vi "Varient_Creator.vi"(8 "error in (no error)":errorcluster) -> (0 "error out":errorcluster)   [LabVIEW 2017]
uses:
  <vilib>/Utility/file.llb/Read Delimited Spreadsheet (string).vi
  <vilib>/Utility/file.llb/Write Delimited Spreadsheet (string).vi
  557cc533-a4ba-4953-a7b5-ba01b5e60265.vi
panel:
  in  "Varient Details":string[][](table)
  in  "Test Resistor":string(combo)
  in  "Magnetic Asyl":string(combo)
  in  "Kinematic Asyl":string(combo)
  in  "CBCT Group":string(combo)
  in  "PMR":string(combo)
  in  "Hausing No":string(combo)
  in  "Delete Button":bool
  in  "Save Button":bool
  in  "Sr  No":u16=1 min=1 max=100 step=1
  in  "HOME":bool
  in  "UPDATE TABLE":bool
  in  "FG CAT No":string(combo)
  # "Varient Creater"
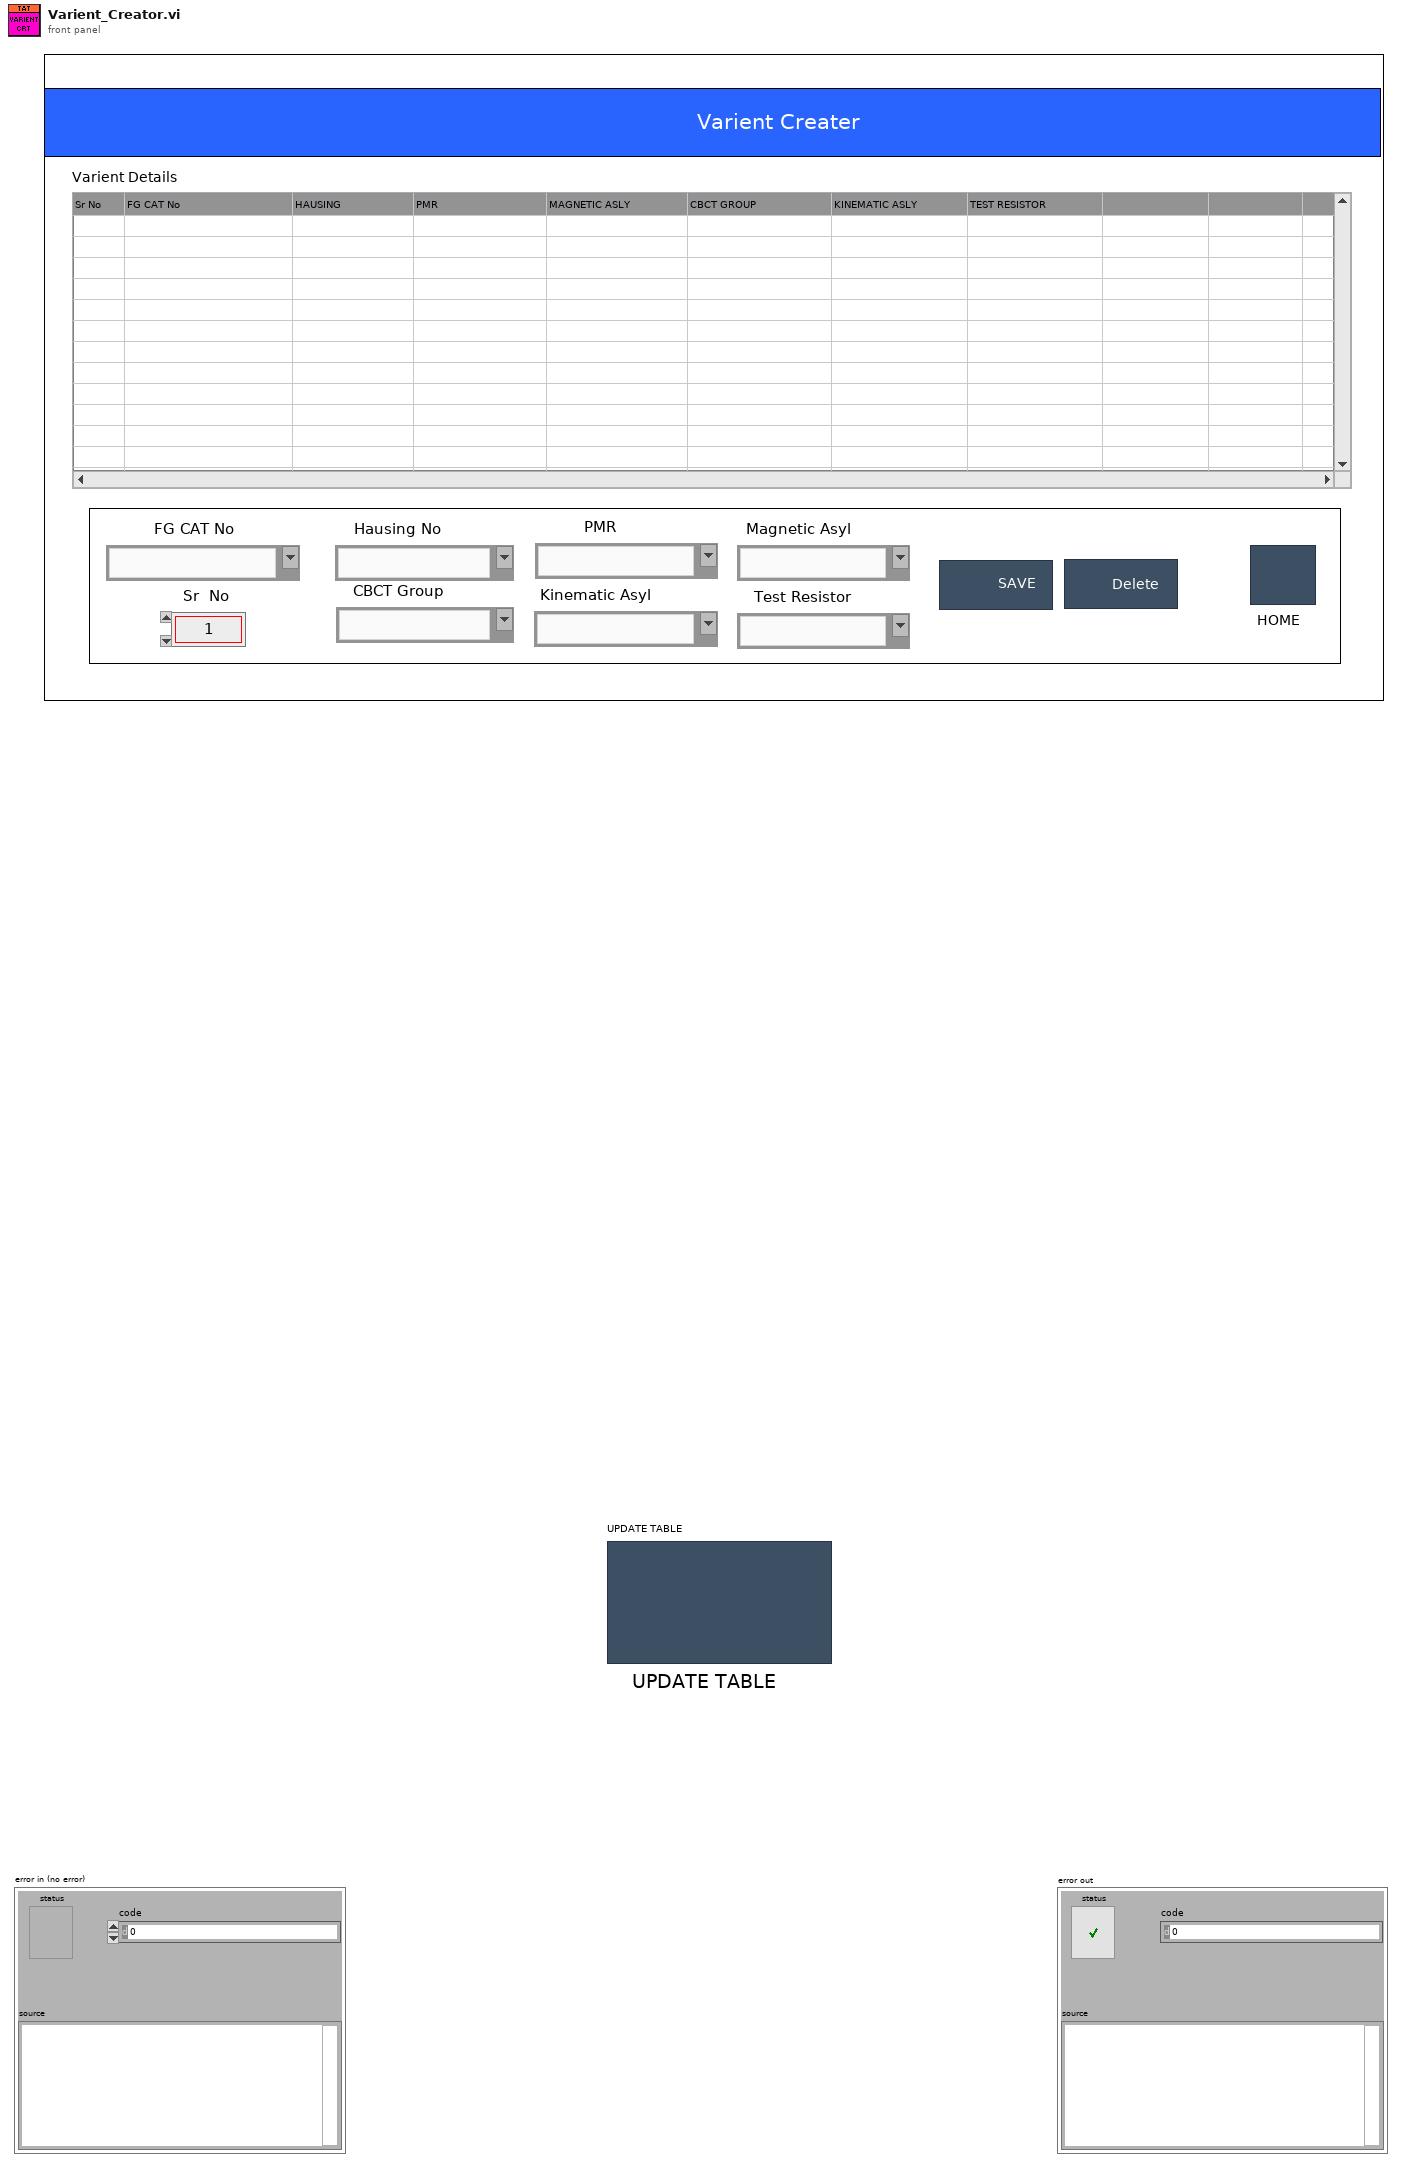
[diagram p1: front panel]
types:
  T1 = enum32{"invalid app kind", "Development System", "Run Time System", "Student Edition", "Embedded LabVIEW", "Evaluation", "Custom"}
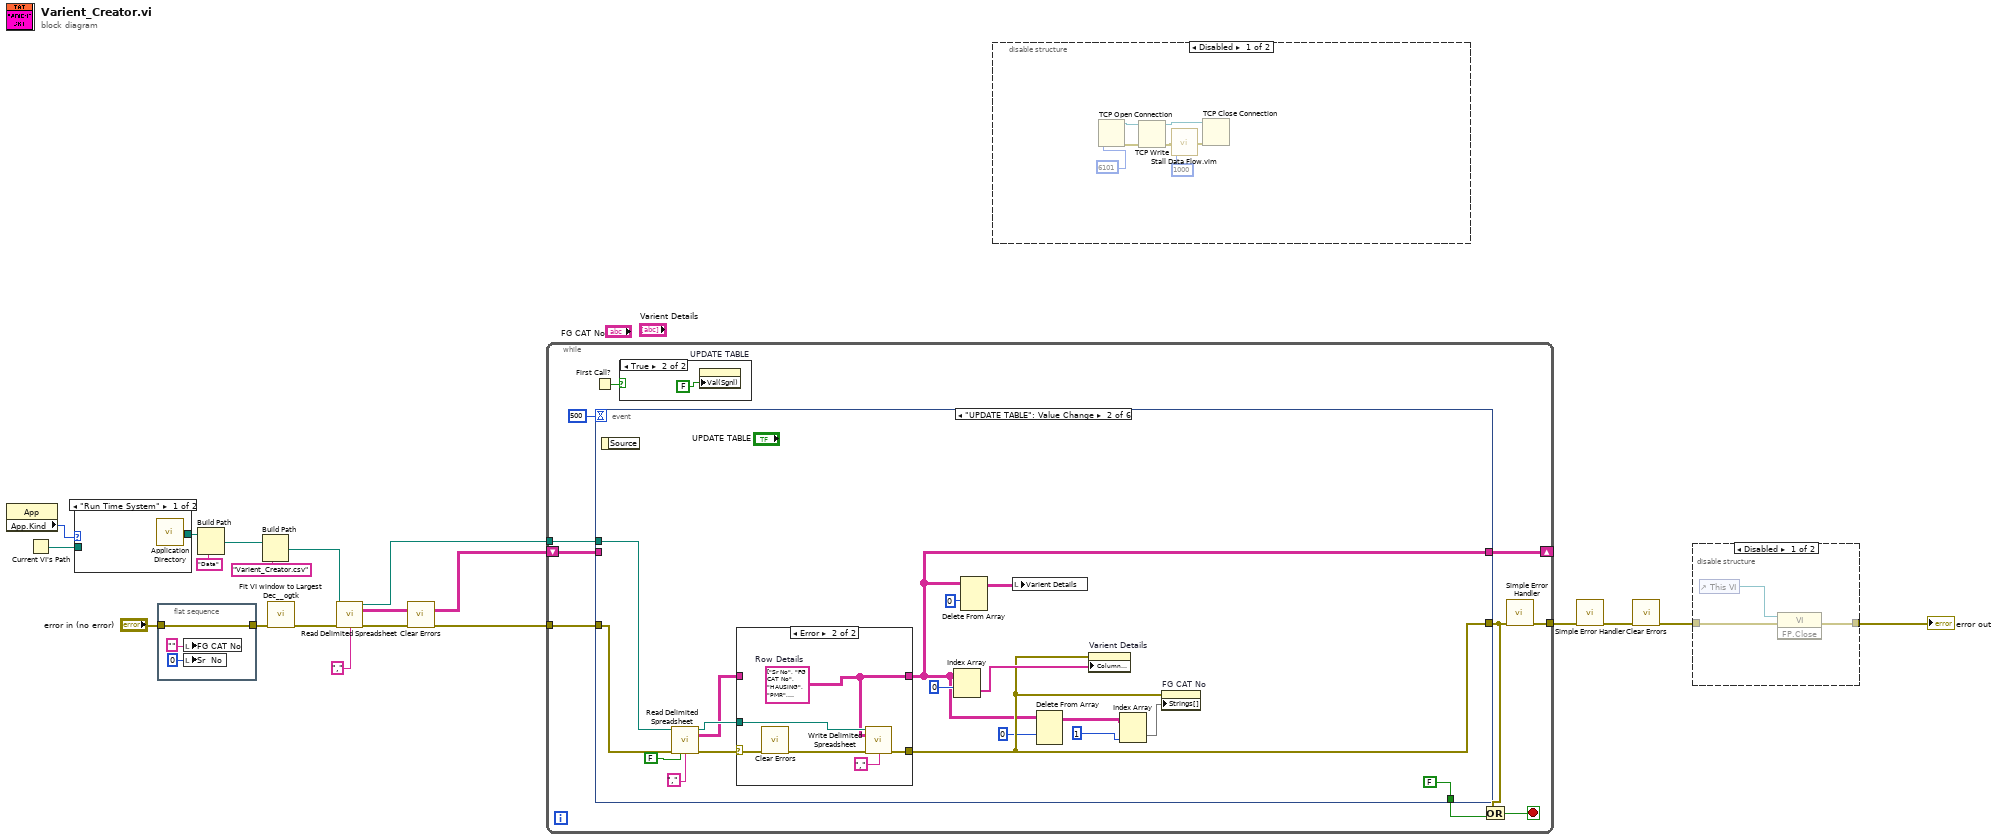
[diagram p0: block diagram]
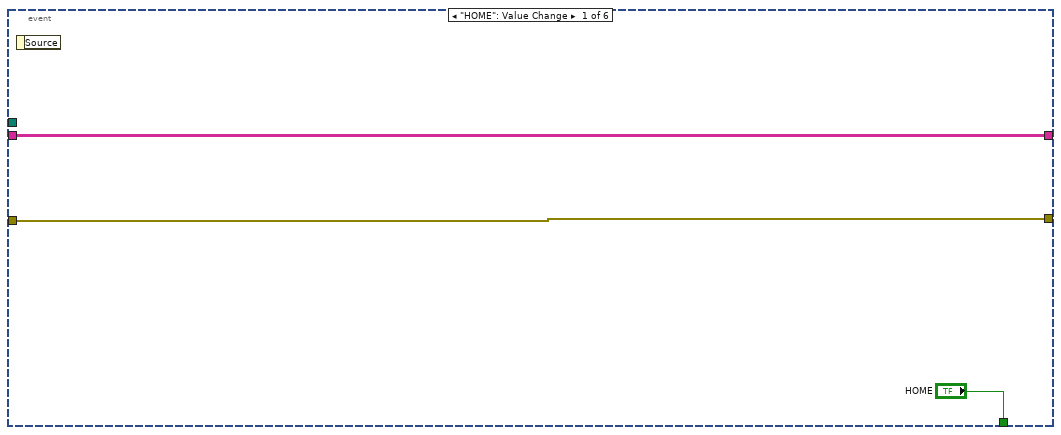
[diagram p3: hidden frame]
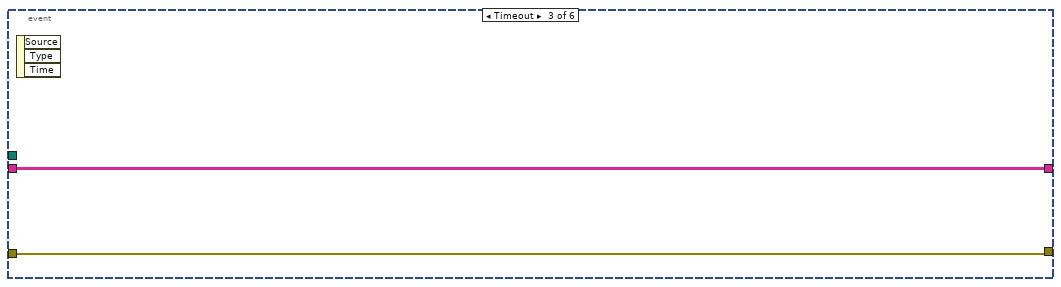
[diagram p5: hidden frame]
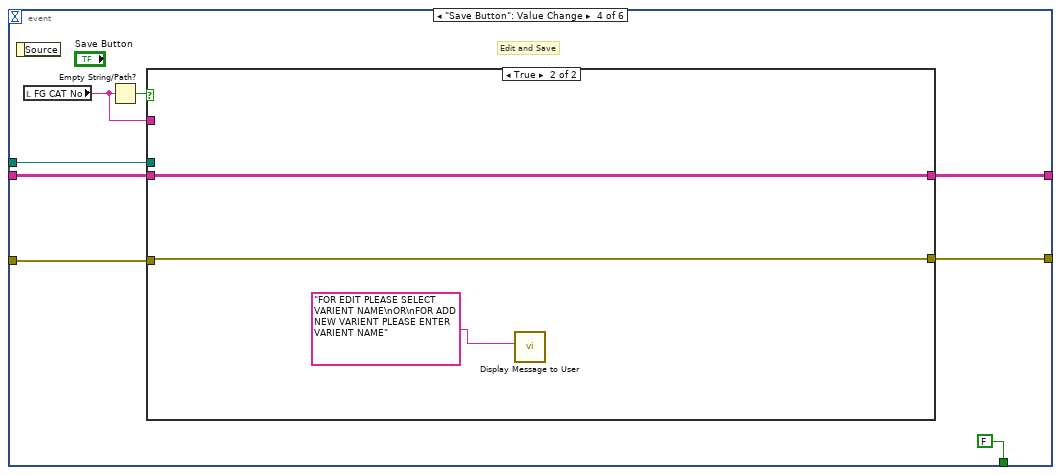
[diagram p6: hidden frame]
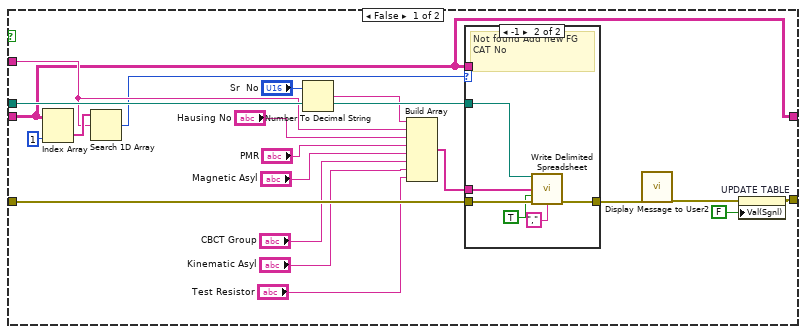
[diagram p7: hidden frame]
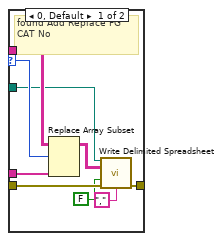
[diagram p8: hidden frame]
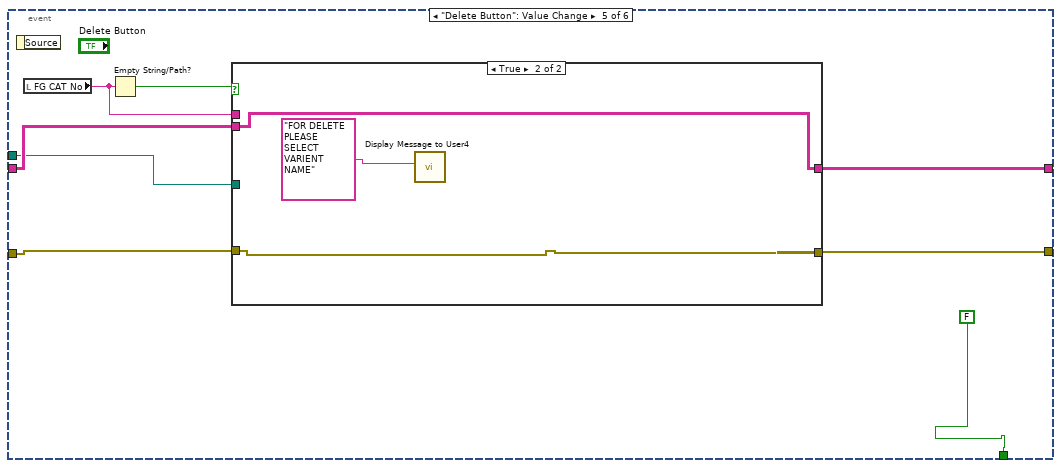
[diagram p9: hidden frame]
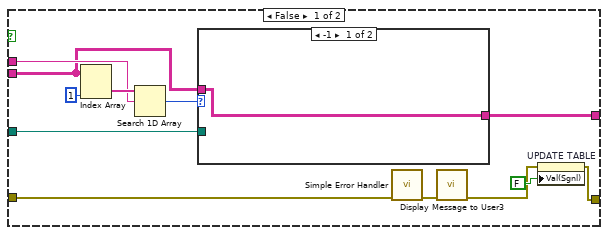
[diagram p10: hidden frame]
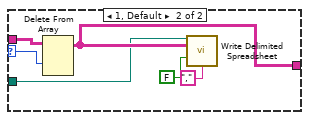
[diagram p11: hidden frame]
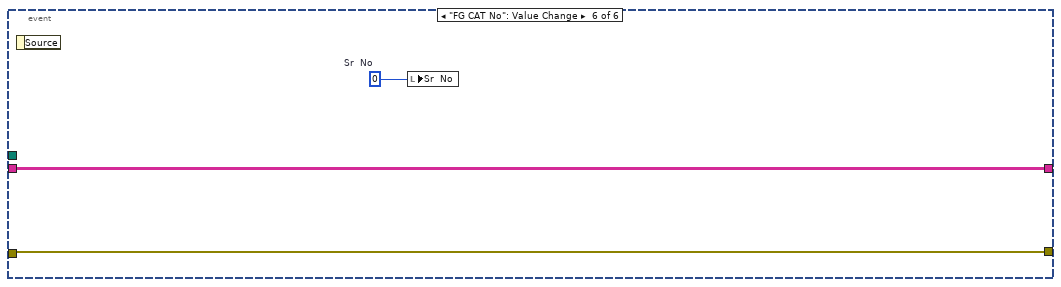
[diagram p12: hidden frame]
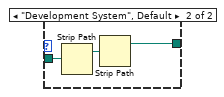
[diagram p15: hidden frame]
diagram:
  n1 = property class="App"() -> ("App.Kind"=w12:T1)  [unwired: 2 in, 2 out]
  n2 = Current VI's Path() -> (path=w13:path)
  n3 = case shown="\"Run Time System\"" w12 {
    tunnel: w13 -> [_ w22]
    tunnel: [w20 w21] -> w9
    frame "Run Time System" {
      n4 = call <vilib>:"Application Directory.vi"() -> ("Application Directory"=w20:path)
    }
    frame "Development System", Default {
      n5 = Strip Path(path=w22) -> (stripped path=w23:path)  [unwired: 1 out]
      n6 = Strip Path(path=w23) -> (stripped path=w21:path)  [unwired: 1 out]
    }
  }
  n7 = flat-sequence {
    tunnel: [w26] -> w14
    tunnel: "error in (no error)" -> [w26]
    frame #0 {
      n8 = local write "FG CAT No"("" ("PART NUMBER")) -> ()
      n9 = local write "Sr  No"(u16 0 ("BATCH SIZE")) -> ()
    }
  }
  n10 = Build Path(base path=w9, name or relative path="Data") -> (appended path=w10:path)
  n11 = Build Path(base path=w10, name or relative path="Varient_Creator.csv") -> (appended path=w1:path)
  n12 = call <userlib>:"Fit VI window to Largest Dec__ogtk.vi"("error in (no error)"=w14) -> ("error out"=w6:errorcluster)  [unwired: 5 in, 1 out]
  n13 = call-poly <vilib>:"Read Delimited Spreadsheet.vi"("file path (dialog if empty)"=w1, "error in (no error)"=w6, "delimiter (\\t)"=",") -> ("new file path (Not A Path if cancelled)"=w7:path, "all rows"=w8:string[][], "error out"=w5:errorcluster)  [unwired: 7 in, 3 out]
  n14 = call <vilib>:"Clear Errors.vi"("error in (no error)"=w5) -> ("error out"=w4:errorcluster)  [unwired: 5 in, 1 out]
  n15 = while {
    tunnel: [w30] -> w16
    tunnel: w4 -> [w33]
    tunnel: w7 -> [w32]
    shift-right: [w29] -> _
    shift-left: w8 -> [w27]
    stop <- w35 stop-if-true
    n16 = First Call?() -> (First Call?: T/F=w34:bool)
    n17 = event shown="[1] \"UPDATE TABLE\": Value Change" {
      selector: _ -> [_ _ _ _ _ _]
      dyn-events: _ -> [_ _ _ _ _ _]
      timeout: 500 -> [_ _ _ _ _ _]
      tunnel: ["HOME" FALSE ("stop") _ FALSE ("stop") FALSE ("stop") _] -> w36
      tunnel: [w38 w47 w66 w73 w118 w144] -> w31
      tunnel: w33 -> [w38 w56 w66 w71 w117 w144]
      tunnel: w27 -> [w37 _ w67 w70 w116 w145]
      tunnel: w32 -> [_ w55 _ w69 w114 _]
      tunnel: [w37 w44 w67 w68 w115 w145] -> w29
      event "HOME": Value Change {
        n18 = event-data() -> ()  [unwired: 1 in, 1 out]
      }
      event "UPDATE TABLE": Value Change {
        n19 = event-data() -> ()  [unwired: 1 in, 1 out]
        n20 = call-poly <vilib>:"Read Delimited Spreadsheet.vi"("file path (dialog if empty)"=w55, "error in (no error)"=w56, "transpose? (F)"=FALSE, "delimiter (\\t)"=",") -> ("new file path (Not A Path if cancelled)"=w52:path, "all rows"=w51:string[][], "error out"=w53:errorcluster)  [unwired: 6 in, 3 out]
        n21 = case shown="Error" w53 {
          selector: w53 -> [w59 w65]
          tunnel: [w59 w63] -> w47
          tunnel: w52 -> [_ w62]
          tunnel: [w58 w60] -> w44
          tunnel: w51 -> [w58 _]
          frame No Error {
          }
          frame Error {
            w60 = string[][] [["Sr No", "FG CAT No", "HAUSING", "PMR", "MAGNETIC ASLY", "CBCT GROUP", "KINEMATIC ASLY", "TEST RESISTOR"]]  # Row Details
            n22 = call <vilib>:"Clear Errors.vi"("error in (no error)"=w65) -> ("error out"=w64:errorcluster)  [unwired: 5 in, 1 out]
            n23 = call-poly <vilib>:"Write Delimited Spreadsheet.vi"("file path (dialog if empty)"=w62, "2D data"=w60, "error in (no error)"=w64, "delimiter (\\t)"=",") -> ("error out"=w63:errorcluster)  [unwired: 10 in, 1 out]
          }
        }
        n24 = Index Array(array=w44, index (row)=0) -> (element=w48:string[])  [unwired: 1 in]
        n25 = Delete From Array(array=w44, index (row)=0) -> (array with subset deleted=w46:string[][])  [unwired: 2 in, 1 out]
        n26 = local write "Varient Details"(w46) -> ()
        n27 = Delete From Array(array=w44, index (row)=0) -> (array with subset deleted=w42:string[][])  [unwired: 2 in, 1 out]
        n28 = property on="Varient Details" class="Tbl (strict)"(error in=w47, "Column Headers[]"=w48) -> ()  [unwired: 1 in, 2 out]
        n29 = Index Array(array=w42, index (col)=1) -> (element=w40:string[])  [unwired: 1 in]
        n30 = property on="FG CAT No" class="CmbBox"(error in=w47, "Strings[]"=w40) -> ()  [unwired: 1 in, 2 out]
      }
      event Timeout {
        n31 = event-data() -> ()  [unwired: 1 in, 3 out]
      }
      event "Save Button": Value Change {
        # "Edit and Save"
        n32 = event-data() -> ()  [unwired: 1 in, 1 out]
        n33 = local read "FG CAT No"() -> (w74:string)
        n34 = Empty String/Path?(string/path=w74) -> (empty?=w72:bool)
        n35 = case shown="True" w72 {
          tunnel: [w94 w112] -> w73
          tunnel: w74 -> [w87 _]
          tunnel: w71 -> [w91 w112]
          tunnel: w70 -> [w81 w111]
          tunnel: w69 -> [w92 _]
          tunnel: [w81 w111] -> w68
          frame False {
            n36 = Index Array(array=w81, index (col)=1) -> (element=w88:string[])  [unwired: 1 in]
            n37 = Search 1D Array(1D array=w88, element=w87) -> (index of element=w82:i32)  [unwired: 1 in]
            n38 = Number To Decimal String(number="Sr  No") -> (decimal integer string=w85:string)  [unwired: 1 in]
            n39 = Build Array(w85, w87, "Hausing No", "PMR", "Magnetic Asyl", "CBCT Group", "Kinematic Asyl", "Test Resistor") -> (w83:string[])
            n40 = case shown="-1" w82 {
              selector: w82 -> [w100 _]
              tunnel: w92 -> [w98 w110]
              tunnel: w91 -> [w103 w109]
              tunnel: [w104 w108] -> w90
              tunnel: w83 -> [w101 w106]
              tunnel: w81 -> [w102 _]
              frame 0, Default {
                # "found Add Replace FG CAT No"
                n41 = Replace Array Subset(array=w102, new element=w101, index (row)=w100) -> (w99:string[][])  [unwired: 1 in]
                n42 = call-poly <vilib>:"Write Delimited Spreadsheet.vi"("file path (dialog if empty)"=w98, "2D data"=w99, "append to file? (new file:F)"=FALSE, "error in (no error)"=w103, "delimiter (\\t)"=",") -> ("error out"=w104:errorcluster)  [unwired: 9 in, 1 out]
              }
              frame -1 {
                # "Not found Add new FG CAT No"
                n43 = call-poly <vilib>:"Write Delimited Spreadsheet.vi"("file path (dialog if empty)"=w110, "1D data"=w106, "append to file? (new file:F)"=TRUE, "error in (no error)"=w109, "delimiter (\\t)"=",") -> ("error out"=w108:errorcluster)  [unwired: 9 in, 1 out]
              }
            }
            n44 = call "Display Message to User2"("error in (no error)"=w90) -> ("error out"=w93:errorcluster)  [unwired: 9 in, 1 out]
            n45 = property on="UPDATE TABLE" class="Bool (strict)"(error in=w93, "Val(Sgnl)"=FALSE) -> (error out=w94:errorcluster)  [unwired: 1 in, 1 out]
          }
          frame True {
            n46 = call "Display Message to User"("Message"="FOR EDIT PLEASE SELECT VARIENT NAME\nOR\nFOR ADD NEW VARIENT PLEASE ENTER VARIENT NAME") -> ()  [unwired: 9 in, 2 out]
          }
        }
      }
      event "Delete Button": Value Change {
        n47 = event-data() -> ()  [unwired: 1 in, 1 out]
        n48 = local read "FG CAT No"() -> (w120:string)
        n49 = Empty String/Path?(string/path=w120) -> (empty?=w119:bool)
        n50 = case shown="True" w119 {
          tunnel: [w132 w142] -> w118
          tunnel: w120 -> [w126 _]
          tunnel: w117 -> [w129 w142]
          tunnel: w116 -> [w124 w141]
          tunnel: [w123 w141] -> w115
          tunnel: w114 -> [w122 _]
          frame False {
            n51 = Index Array(array=w124, index (col)=1) -> (element=w127:string[])  [unwired: 1 in]
            n52 = Search 1D Array(1D array=w127, element=w126) -> (index of element=w125:i32)  [unwired: 1 in]
            n53 = case shown="-1" w125 {
              selector: w125 -> [_ w139]
              tunnel: w124 -> [w134 w140]
              tunnel: [w134 w136] -> w123
              tunnel: w122 -> [_ w135]
              frame -1 {
              }
              frame 1, Default {
                n54 = Delete From Array(array=w140, index (row)=w139) -> (array with subset deleted=w136:string[][])  [unwired: 2 in, 1 out]
                n55 = call-poly <vilib>:"Write Delimited Spreadsheet.vi"("file path (dialog if empty)"=w135, "2D data"=w136, "append to file? (new file:F)"=FALSE, "delimiter (\\t)"=",") -> ()  [unwired: 10 in, 2 out]
              }
            }
            n56 = call <vilib>:"Simple Error Handler.vi"("error in (no error)"=w129) -> ("error out"=w131:errorcluster)  [unwired: 4 in, 4 out]
            n57 = call "Display Message to User3"("error in (no error)"=w131) -> ("error out"=w130:errorcluster)  [unwired: 9 in, 1 out]
            n58 = property on="UPDATE TABLE" class="Bool (strict)"(error in=w130, "Val(Sgnl)"=FALSE) -> (error out=w132:errorcluster)  [unwired: 1 in, 1 out]
          }
          frame True {
            n59 = call "Display Message to User4"("Message"="FOR DELETE PLEASE SELECT VARIENT NAME") -> ()  [unwired: 9 in, 2 out]
          }
        }
      }
      event "FG CAT No": Value Change {
        w146 = u16 0  # Sr  No
        n60 = event-data() -> ()  [unwired: 1 in, 1 out]
        n61 = local write "Sr  No"(w146) -> ()
      }
    }
    n62 = case shown="True" w34 {
      frame False {
      }
      frame True {
        n63 = property on="UPDATE TABLE" class="Bool (strict)"("Val(Sgnl)"=FALSE) -> ()  [unwired: 2 in, 2 out]
      }
    }
    n64 = Or(x=w31, y=w36) -> (x .or. y?=w35:bool)
    n65 = call <vilib>:"Simple Error Handler.vi"("error in (no error)"=w31) -> ("error out"=w30:errorcluster)  [unwired: 4 in, 4 out]
  }
  n66 = disable-structure shown="Disabled" {
    frame Disabled {
      n67 = TCP Open Connection(remote port or service name=u16 6101) -> (connection ID=w153:refnum<k5>, error out=w152:errorcluster)  [unwired: 4 in]
      n68 = TCP Write(connection ID=w153, error in (no error)=w152) -> (connection ID out=w155:refnum<k5>, error out=w151:errorcluster)  [unwired: 2 in, 1 out]
      n69 = call "Stall Data Flow.vim"("value in"=w151, "milliseconds to wait"=u32 1000) -> ("value out"=w154:errorcluster)  [unwired: 1 out]
      n70 = TCP Close Connection(connection ID=w155, error in (no error)=w154) -> (error out=w148:errorcluster)  [unwired: 1 in, 1 out]
    }
    frame Enabled {
    }
  }
  n71 = call <vilib>:"Simple Error Handler.vi"("error in (no error)"=w16) -> ("error out"=w19:errorcluster)  [unwired: 4 in, 4 out]
  n72 = call <vilib>:"Clear Errors.vi"("error in (no error)"=w19) -> ("error out"=w18:errorcluster)  [unwired: 5 in, 1 out]
  n73 = disable-structure shown="Disabled" {
    disable-tunnel: w18 -> [w158 w159]
    disable-tunnel: [w157 w159] -> w17
    frame Disabled {
      n74 = control-ref of="This VI"() -> (w156:refnum<vi>)
      n75 = invoke class="VI" method="FP.Close"(reference=w156, error in=w158) -> (error out=w157:errorcluster)  [unwired: 1 in, 2 out]
    }
    frame Enabled {
    }
  }
  "error out" <- w17
